vi "StartCapture.vi"(8 "error in (no error)":errorcluster, 10 "Continuous":bool, 11 "HamaCam in":refnum<class "HamaCam.lvclass">) -> (0 "error out":errorcluster, 3 "HamaCam out":refnum<class "HamaCam.lvclass">)   [LabVIEW 2023, in "HamaCam.lvlib" / "HamaCam.lvclass"]
uses:
  HamaCam.lvclass
  HamaCam.lvclass/HamaCam.ctl
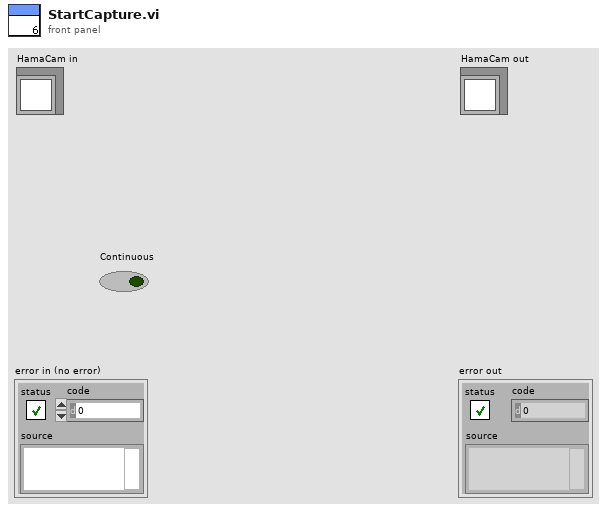
[diagram p1: front panel]
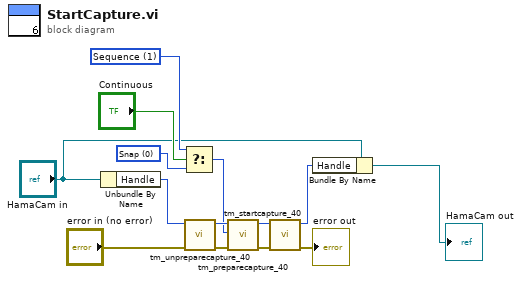
[diagram p0: block diagram]
diagram:
  w7 = 0 items=["Snap", "Sequence"] ("Capture mode")
  w10 = 1 items=["Snap", "Sequence"] ("Capture mode")
  n1 = Unbundle By Name("HamaCam in") -> ("Handle"=w6:u32)
  n2 = Select(t=w10, s="Continuous", f=w7) -> (s? t:f=w9:i32)
  n3 = call "tm_unpreparecapture_40.vi"("error in (no error)"="error in (no error)", "Handle in"=w6) -> ("error out"=w12:errorcluster, "Handle out"=w11:u32)  [unwired: 8 in]
  n4 = call "tm_preparecapture_40.vi"("error in (no error)"=w12, "Capture mode"=w9, "Handle in"=w11) -> ("error out"=w13:errorcluster, "Handle out"=w14:u32)  [unwired: 5 in, 2 out]
  n5 = call "tm_startcapture_40.vi"("error in (no error)"=w13, "Handle in"=w14) -> ("error out"=→"error out":errorcluster, "Handle out"=w4:u32)  [unwired: 8 in]
  n6 = Bundle By Name(cluster="HamaCam in", "Handle"=w4) -> (→"HamaCam out":refnum<class "HamaCam.lvclass">)
